vi "Add.vi"(1 "x":sgl, 2 "y":sgl, 4 "Adder2":refnum<class "Adder2.lvclass">) -> (6 "x+y":sgl)   [LabVIEW 2017, in "Adder2.lvclass"]
uses:
  Adder2.lvclass
  Adder.lvclass
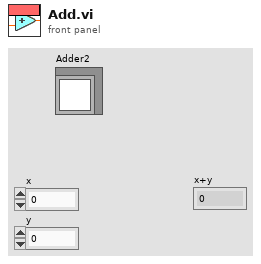
[diagram p1: front panel]
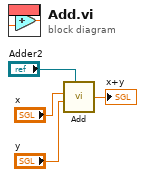
[diagram p0: block diagram]
diagram:
  n1 = call-parent "Add.vi"("x"="x", "y"="y", "Adder"="Adder2") -> ("x+y"=→"x+y":sgl)  [unwired: 4 in]
